vi "Shipping Position.vi"(6 "Shipping":dbl=200.0 format="%#_13g", 7 "Model Name":T1, 8 "Error In":errorcluster, 9 "Intialize?":bool=TRUE, 10 "Inputs":T2) -> (0 "error out":errorcluster, 1 "Completed":bool, 3 "Results":cluster{"Shipping Position":dbl}, 4 "Status":cluster{"Status":string, "Elapsed Time":dbl})   [LabVIEW 2017]
doc: "v0.1:\n- Bypass sensor 1"
uses:
  controls/FGV DO.ctl
  controls/Shipping Position.ctl
  controls/All Inputs.ctl
  controls/Model Name.ctl
  controls/SACB DI.ctl
panel:
  in  "Wait for Motor Stop":u32=1000
  in  "Delay (for Rest)":u32=500
  in  "Timeout (ms)":u32=15000
  # "Inputs"
  # "Variables"
  # "Outputs"
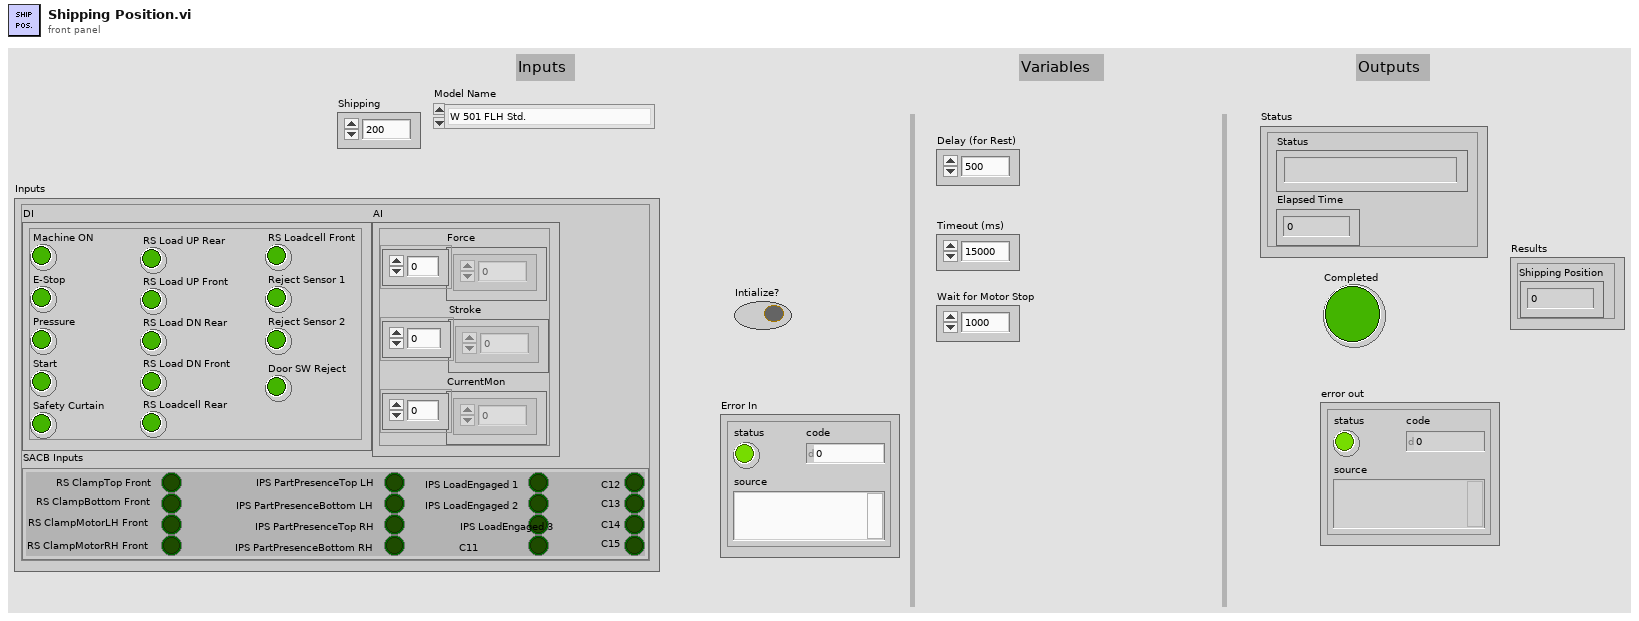
[diagram p1: front panel]
types:
  T1 = typedef "Model Name.ctl" = enum16{"W 501 FLH Std.", "W 501 FRH Std.", "W 601 FR RH Std", "W 601 FR LH Std", "W 601 RR RH Std", "W 601 RR LH Std", "W 601 FR RH AP", "W 601 FR LH AP", "W 601 RR RH AP", "W 601 RR LH AP"}
  T2 = typedef "All Inputs.ctl" = cluster{"DI":cluster{"Machine ON":bool, "E-Stop":bool, "Pressure":bool, "Start":bool, "Safety Curtain":bool, "RS Load UP Rear":bool, "RS Load UP Front":bool, "RS Load DN Rear":bool, "RS Load DN Front":bool, "RS Loadcell Rear":bool, "RS Loadcell Front":bool, "Reject Sensor 1":bool, "Reject Sensor 2":bool, "Door SW Reject":bool}, "AI":cluster{"Force":dbl[], "Stroke":dbl[], "CurrentMon":dbl[]}, "SACB Inputs":T3}
  T3 = typedef "SACB DI.ctl" = cluster{"RS ClampTop Front":bool, "RS ClampBottom Front":bool, "RS ClampMotorLH Front":bool, "RS ClampMotorRH Front":bool, "IPS PartPresenceTop LH":bool, "IPS PartPresenceBottom LH":bool, "IPS PartPresenceTop RH":bool, "IPS PartPresenceBottom RH":bool, "IPS LoadEngaged 1":bool, "IPS LoadEngaged 2":bool, "IPS LoadEngaged 3":bool, "C11":bool, "C12":bool, "C13":bool, "C14":bool, "C15":bool}
  T4 = typedef "Shipping Position.ctl" = enum16{"Initialize", "Set Loading", "Go UP", "Wait for Shipping Position", "Short Terminals", "Wait for Motor Stop", "Turn Off Supply", "Check Shipping Position", "Remove Loading", "Wait for Rest", "Done", "Error"}
  T5 = typedef "FGV DO.ctl" = enum16{"Initialize", "Start Task", "Clamping", "Load CYL", "Contactors", "Loadcell CYL", "BSL", "Read DO", "Clear Tasks", "Clear Task"}
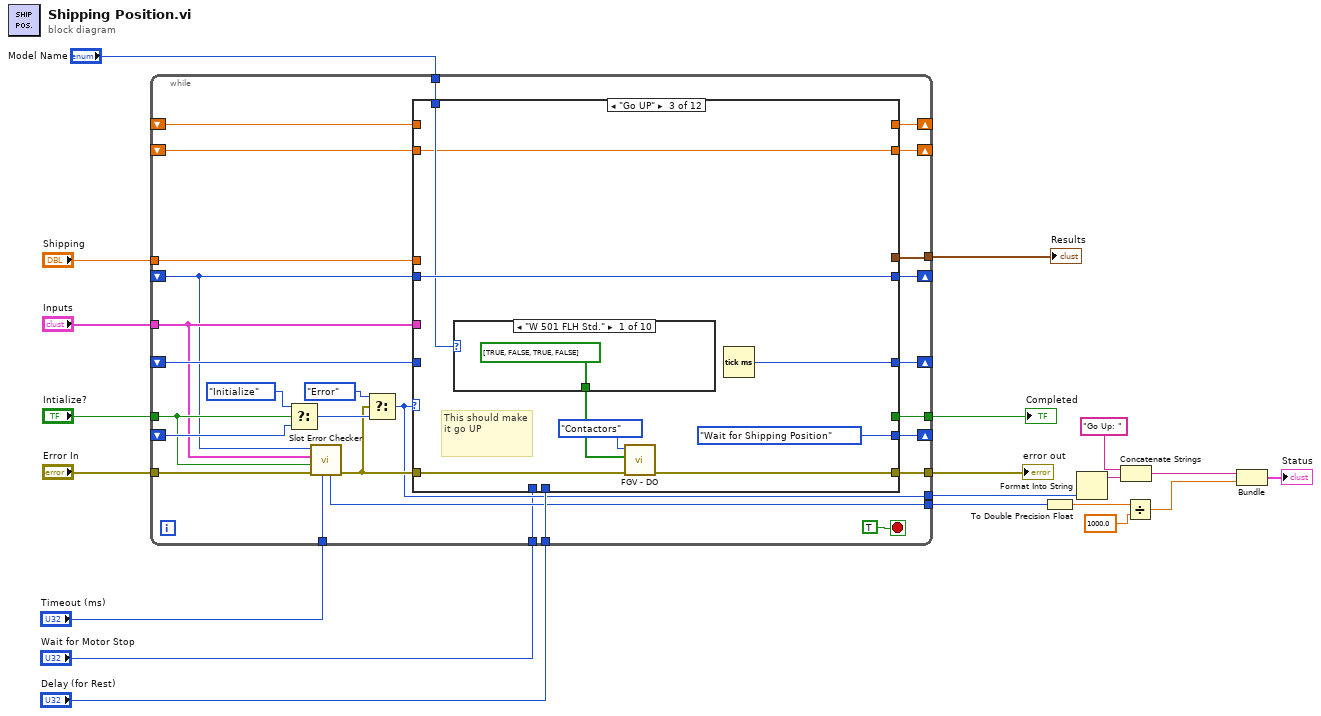
[diagram p0: block diagram]
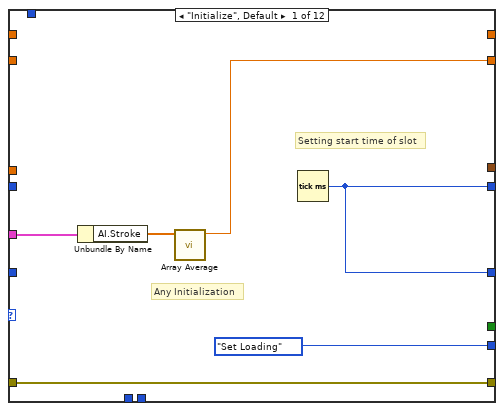
[diagram p2: hidden frame]
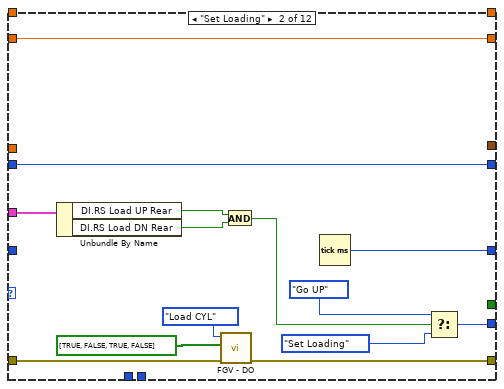
[diagram p3: hidden frame]
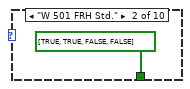
[diagram p4: hidden frame]
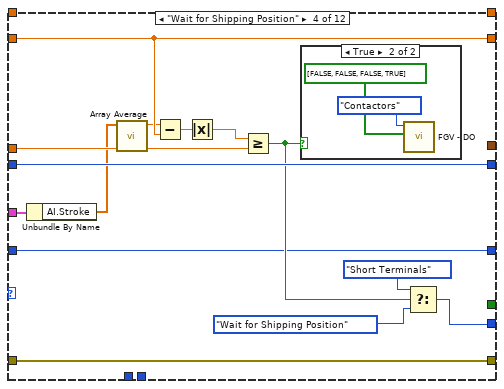
[diagram p13: hidden frame]
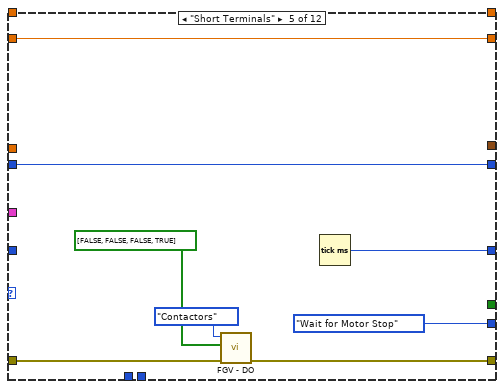
[diagram p15: hidden frame]
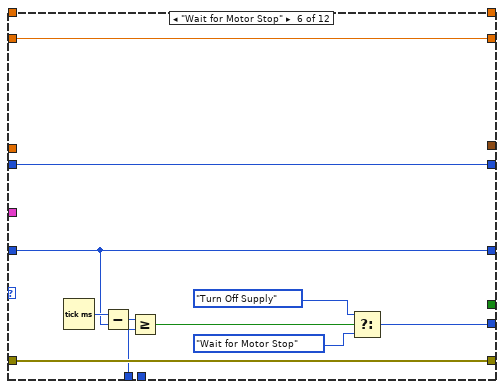
[diagram p16: hidden frame]
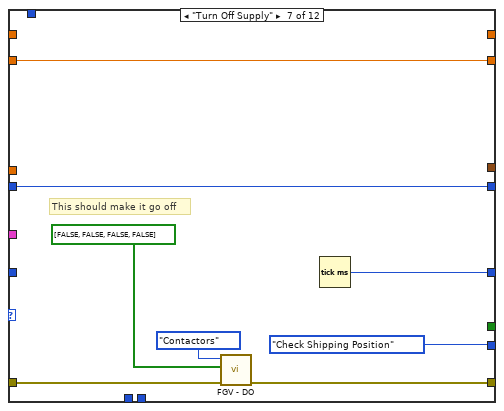
[diagram p17: hidden frame]
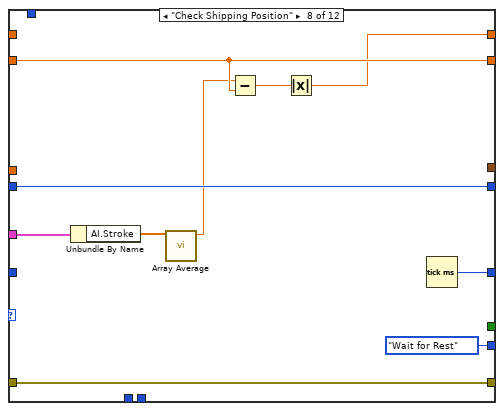
[diagram p18: hidden frame]
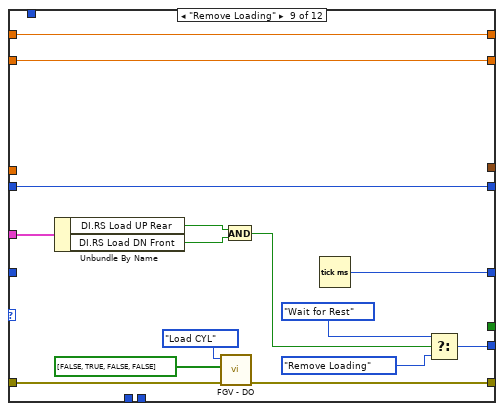
[diagram p19: hidden frame]
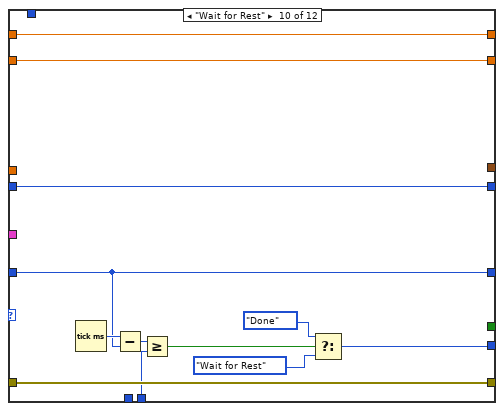
[diagram p20: hidden frame]
diagram:
  n1 = while {
    tunnel: "Intialize?" -> [w38]
    shift-right: [w45] -> _
    shift-left: _ -> [w47]
    shift-right: [w44] -> _
    shift-left: _ -> [w43]
    tunnel: "Error In" -> [w39]
    tunnel: [w42] -> w20
    tunnel: [w41] -> w19
    tunnel: "Inputs" -> [w37]
    shift-right: [w40] -> _
    shift-left: _ -> [w36]
    tunnel: "Delay (for Rest)" -> [w32]
    tunnel: "Timeout (ms)" -> [w31]
    tunnel: "Model Name" -> [w30]
    shift-right: [w29] -> _
    shift-left: _ -> [w28]
    tunnel: [w27] -> w12
    tunnel: [w26] -> w4
    tunnel: [w25] -> w3
    tunnel: "Wait for Motor Stop" -> [w24]
    shift-right: [w23] -> _
    shift-left: _ -> [w22]
    tunnel: "Shipping" -> [w21]
    stop <- TRUE stop-if-true
    n2 = Select(t=Shipping_Position."Initialize", s=w38, f=w47) -> (s? t:f=w35:T4)
    n3 = call "Slot Error Checker.vi"("Timeout (ms)"=w31, "error in (no error)"=w39, "Intialize?"=w38, "Inputs"=w37, "start time"=w36) -> ("error out"=w34:errorcluster, "Slot Time"=w26:u32)  [unwired: 5 in]
    n4 = Select(t=Shipping_Position."Error", s=w34, f=w35) -> (s? t:f=w25:T4)
    n5 = case shown="\"Go UP\"" w25 {
      tunnel: [Shipping_Position."Set Loading" w58 Shipping_Position."Wait for Shipping Position" w90 Shipping_Position."Wait for Motor Stop" w111 Shipping_Position."Check Shipping Position" Shipping_Position."Wait for Rest" w137 w156 Shipping_Position."Done" Shipping_Position."Done"] -> w45
      tunnel: [w52 w63 w71 w87 w98 w113 w117 w130 w142 w158 _ _] -> w44
      tunnel: w43 -> [_ _ _ w87 _ w113 _ _ _ w158 _ _]
      tunnel: w34 -> [w53 w68 w77 w92 w103 w109 w122 w131 w147 w154 w166 w173]
      tunnel: [w53 w67 w76 w92 w102 w109 w121 w131 w146 w154 w166 w173] -> w42
      tunnel: [_ _ _ _ _ _ _ _ _ _ w165 TRUE ("Completed")] -> w41
      tunnel: w37 -> [w51 w61 _ w84 _ _ _ w128 w140 _ _ _]
      tunnel: [w52 w64 w73 w93 w99 w106 w116 w132 w143 w151 w164 w170] -> w40
      tunnel: w36 -> [_ w64 w73 w93 w99 w106 w116 w132 w143 w151 w164 w170]
      tunnel: w32 -> [_ _ _ _ _ _ _ _ _ w150 _ _]
      tunnel: w30 -> [_ _ w72 _ _ _ _ _ _ _ _ _]
      tunnel: [_ _ _ _ _ _ _ w123 w133 w149 _ _] -> w29
      tunnel: w28 -> [_ _ _ _ _ _ _ _ w133 w149 w162 _]
      tunnel: [_ _ _ _ _ _ _ _ _ _ w163 _] -> w27
      tunnel: w24 -> [_ _ _ _ _ w105 _ _ _ _ _ _]
      tunnel: [w49 w62 w69 w83 w96 w104 w115 w126 w141 w148 w160 _] -> w23
      tunnel: w22 -> [_ w62 w69 w83 w96 w104 w115 w126 w141 w148 w160 _]
      tunnel: w21 -> [_ _ _ w86 _ _ _ _ _ _ _ _]
      frame "Initialize", Default {
        # "Setting start time of slot"
        # "Any Initialization"
        n6 = Unbundle By Name(w51) -> ("AI.Stroke"=w50:dbl[])
        n7 = call "Array Average.vi"("data"=w50) -> ("Numeric"=w49:dbl)  [unwired: 10 in]
        n8 = Tick Count (ms)() -> (millisecond timer value=w52:u32)
      }
      frame "Set Loading" {
        n9 = Unbundle By Name(w61) -> ("DI.RS Load UP Rear"=w60:bool, "DI.RS Load DN Rear"=w59:bool)
        n10 = call "FGV - DO.vi"("error in"=w68, "Digital Outs"=bool[] [TRUE, FALSE, TRUE, FALSE], "State"=FGV_DO."Load CYL") -> ("error out"=w67:errorcluster)  [unwired: 7 in, 1 out]
        n11 = And(x=w60, y=w59) -> (x .and. y?=w55:bool)
        n12 = Tick Count (ms)() -> (millisecond timer value=w63:u32)
        n13 = Select(t=Shipping_Position."Go UP", s=w55, f=Shipping_Position."Set Loading") -> (s? t:f=w58:T4)
      }
      frame "Go UP" {
        # "This should make it go UP"
        n14 = case shown="\"W 501 FLH Std.\"" w72 {
          tunnel: [bool[] [TRUE, FALSE, TRUE, FALSE] ("Digital Outs") bool[] [TRUE, TRUE, FALSE, FALSE] ("Digital Outs") _ _ _ _ _ _ _ _] -> w74
          frame "W 501 FLH Std." {
          }
          frame "W 501 FRH Std." {
          }
          frame "W 601 FR RH Std" {
          }
          frame "W 601 FR LH Std" {
          }
          frame "W 601 RR RH Std" {
          }
          frame "W 601 RR LH Std" {
          }
          frame "W 601 FR RH AP" {
          }
          frame "W 601 FR LH AP" {
          }
          frame "W 601 RR RH AP" {
          }
          frame "W 601 RR LH AP" {
          }
        }
        n15 = call "FGV - DO.vi"("error in"=w77, "Digital Outs"=w74, "State"=FGV_DO."Contactors") -> ("error out"=w76:errorcluster)  [unwired: 7 in, 1 out]
        n16 = Tick Count (ms)() -> (millisecond timer value=w71:u32)
      }
      frame "Wait for Shipping Position" {
        n17 = Unbundle By Name(w84) -> ("AI.Stroke"=w82:dbl[])
        n18 = call "Array Average.vi"("data"=w82) -> ("Numeric"=w81:dbl)  [unwired: 10 in]
        n19 = Subtract(x=w81, y=w83) -> (x-y=w85:dbl)
        n20 = Absolute Value(x=w85) -> (abs(x)=w80:dbl)
        n21 = Greater Or Equal?(x=w80, y=w86) -> (x >= y?=w88:bool)
        n22 = case shown="True" w88 {
          frame False {
          }
          frame True {
            n23 = call "FGV - DO.vi"("Digital Outs"=bool[] [FALSE, FALSE, FALSE, TRUE], "State"=FGV_DO."Contactors") -> ()  [unwired: 8 in, 2 out]
          }
        }
        n24 = Select(t=Shipping_Position."Short Terminals", s=w88, f=Shipping_Position."Wait for Shipping Position") -> (s? t:f=w90:T4)
      }
      frame "Short Terminals" {
        n25 = call "FGV - DO.vi"("error in"=w103, "Digital Outs"=bool[] [FALSE, FALSE, FALSE, TRUE], "State"=FGV_DO."Contactors") -> ("error out"=w102:errorcluster)  [unwired: 7 in, 1 out]
        n26 = Tick Count (ms)() -> (millisecond timer value=w98:u32)
      }
      frame "Wait for Motor Stop" {
        n27 = Tick Count (ms)() -> (millisecond timer value=w114:u32)
        n28 = Subtract(x=w114, y=w113) -> (x-y=w112:u32)
        n29 = Greater Or Equal?(x=w112, y=w105) -> (x >= y?=w110:bool)
        n30 = Select(t=Shipping_Position."Turn Off Supply", s=w110, f=Shipping_Position."Wait for Motor Stop") -> (s? t:f=w111:T4)
      }
      frame "Turn Off Supply" {
        # "This should make it go off"
        n31 = call "FGV - DO.vi"("error in"=w122, "Digital Outs"=bool[] [FALSE, FALSE, FALSE, FALSE], "State"=FGV_DO."Contactors") -> ("error out"=w121:errorcluster)  [unwired: 7 in, 1 out]
        n32 = Tick Count (ms)() -> (millisecond timer value=w117:u32)
      }
      frame "Check Shipping Position" {
        n33 = Unbundle By Name(w128) -> ("AI.Stroke"=w127:dbl[])
        n34 = call "Array Average.vi"("data"=w127) -> ("Numeric"=w125:dbl)  [unwired: 10 in]
        n35 = Subtract(x=w125, y=w126) -> (x-y=w124:dbl)
        n36 = Absolute Value(x=w124) -> (abs(x)=w123:dbl)
        n37 = Tick Count (ms)() -> (millisecond timer value=w130:u32)
      }
      frame "Remove Loading" {
        n38 = Unbundle By Name(w140) -> ("DI.RS Load UP Rear"=w139:bool, "DI.RS Load DN Front"=w138:bool)
        n39 = call "FGV - DO.vi"("error in"=w147, "Digital Outs"=bool[] [FALSE, TRUE, FALSE, FALSE], "State"=FGV_DO."Load CYL") -> ("error out"=w146:errorcluster)  [unwired: 7 in, 1 out]
        n40 = And(x=w139, y=w138) -> (x .and. y?=w134:bool)
        n41 = Tick Count (ms)() -> (millisecond timer value=w142:u32)
        n42 = Select(t=Shipping_Position."Wait for Rest", s=w134, f=Shipping_Position."Remove Loading") -> (s? t:f=w137:T4)
      }
      frame "Wait for Rest" {
        n43 = Tick Count (ms)() -> (millisecond timer value=w159:u32)
        n44 = Subtract(x=w159, y=w158) -> (x-y=w157:u32)
        n45 = Greater Or Equal?(x=w157, y=w150) -> (x >= y?=w155:bool)
        n46 = Select(t=Shipping_Position."Done", s=w155, f=Shipping_Position."Wait for Rest") -> (s? t:f=w156:T4)
      }
      frame "Done" {
        w165 = TRUE  # Completed
        n47 = Bundle(cluster=cluster{"PES_Shipping_RLH_Position":dbl} {"PES_Shipping_RLH_Position"=0.0}, "PES_Shipping_RLH_Position"=w162) -> (w163:cluster{"PES_Shipping_RLH_Position":dbl})
      }
      frame "Error" {
        w168 = T5[] [enum."Clamping", enum."Load CYL", enum."Contactors"] items=["Initialize", "Start Task", "Clamping", "Load CYL", "Contactors", "Loadcell CYL", "BSL", "Read DO", "Clear Tasks", "Clear Task"]
        n48 = for {
          tunnel: w168 -> [w175] mode=indexing
          tunnel: bool[] [FALSE, FALSE, FALSE, FALSE] ("Digital Outs") -> [w174]
          n49 = call "FGV - DO.vi"("Digital Outs"=w174, "State"=w175) -> ()  [unwired: 8 in, 2 out]
        }
      }
    }
  }
  "error out" <- w20
  "Completed" <- w19
  "Results" <- w12
  n50 = To Double Precision Float(number=w4) -> (double precision float=w9:dbl)
  n51 = Format Into String(w3) -> (resulting string=w11:string)  [unwired: 3 in, 1 out]
  n52 = Concatenate Strings("Go Up: ", w11) -> (w7:string)
  n53 = Divide(x=w9, y=1000.0) -> (x/y=w6:dbl)
  n54 = Bundle(w7, w6) -> (→"Status":cluster{string, dbl})  [unwired: 1 in]
